vi "After Launch Init Core.vi"(8 "error in (no error)":errorcluster, 11 "CS++DeviceActor in":refnum<class "CS++DeviceActor.lvclass">) -> (0 "error out":errorcluster, 3 "CS++DeviceActor out":refnum<class "CS++DeviceActor.lvclass">)   [LabVIEW 2014, in "CS++DeviceActor.lvlib" / "CS++DeviceActor.lvclass"]
doc: "Use <b>Pre Launch init.vi</b> method for sanity checks that are supposed to prevent the actor from launching if they fail. Use <B>this</B> method instead to initialize this actor when it has been activated. A corresponding high priority message will become dispatched before the <B>Actor Core.vi</b> is called.\n\n<b>Derived classed should call the parent methode first</b> and their own initialization code after.\n\nRefer also to the ongoing discussion at https://decibel.ni.com/content/message/57394#57394."
uses:
  CS++DeviceActor.lvclass
  CS++DeviceActor.lvclass/CS++DeviceActor.ctl
  CS++BaseActor/CS++BaseActor.lvclass/CS++BaseActor.ctl
  <vilib>/ActorFramework/Actor/Actor.lvclass/Actor.ctl
  <vilib>/ActorFramework/Message Enqueuer/Message Enqueuer.lvclass/Message Enqueuer.ctl
  CS++DeviceActor Messages/Initialize Device Msg/Initialize Device Msg.lvclass/Initialize Device Msg.ctl
  CS++BaseActor Messages/Launch Associated GUI Msg/Launch Associated GUI Msg.lvclass/Launch Associated GUI Msg.ctl
  <vilib>/ActorFramework/Message Enqueuer/Enqueue.vi
  <vilib>/ActorFramework/Message Enqueuer/Init from Existing Queue.vi
  <vilib>/ActorFramework/Message Priority Queue/Priority Enqueue.vi
  CS++BaseActor/CS++BaseActor.lvclass
  CS++BaseActor Messages/Launch Associated GUI Msg/Launch Associated GUI Msg.lvclass
  CS++DeviceActor Messages/Selftest Device Msg/Selftest Device Msg.lvclass
  CS++DeviceActor Messages/Initialize Device Msg/Initialize Device Msg.lvclass
  <vilib>/ActorFramework/Message Enqueuer/Message Enqueuer.lvclass
  <vilib>/ActorFramework/Actor/Actor.lvclass
  Classes/CS++ProcessVariables/PVConnection/PVConnection.lvclass
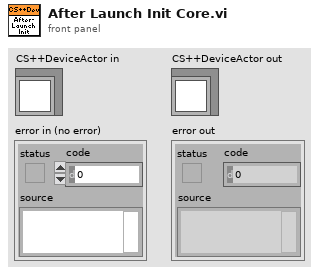
[diagram p1: front panel]
types:
  T1 = cluster{"Write Access":enum8{"Allowed", "Required", "None"}, "Read Access":enum8{"Allowed", "Required", "None"}}
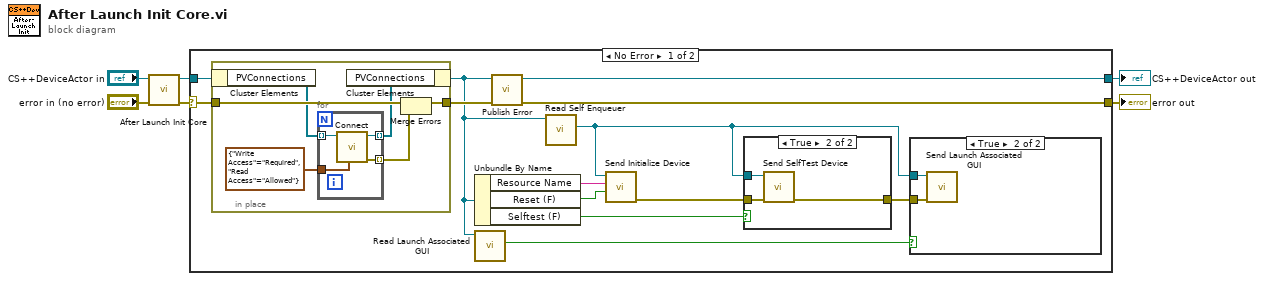
[diagram p0: block diagram]
diagram:
  n1 = call-parent "After Launch Init Core.vi"("error in (no error)"="error in (no error)", "CS++BaseActor in"="CS++DeviceActor in") -> ("error out"=w1:errorcluster, "CS++BaseActor out"=w3:refnum<class "CS++DeviceActor.lvclass">)  [unwired: 8 in]
  n2 = case shown="No Error" w1 {
    selector: w1 -> [w7 w36]
    tunnel: w3 -> [w8 w37]
    tunnel: [w11 w36] -> w6
    tunnel: [w10 w37] -> w5
    frame No Error {
      n3 = in-place {
        in-place-border: [w25] -> w18
        in-place-border: w7 -> [w24]
        n4 = in-place-cluster #1(w8) -> ("PVConnections"=w21:refnum<class "PVConnection.lvclass">[])
        n5 = for {
          tunnel: w21 -> [w29] mode=indexing
          tunnel: [w28] -> w20 mode=indexing
          tunnel: T1 {"Write Access"=enum."Required", "Read Access"=enum."Allowed"} ("Access") -> [w27]
          tunnel: [w26] -> w22 mode=indexing
          n6 = call "Connect.vi"("Access (R/W allowed)"=w27, "PVConnection in"=w29) -> ("error out"=w26:errorcluster, "PVConnection out"=w28:refnum<class "PVConnection.lvclass">)  [unwired: 8 in]
        }
        n7 = in-place-cluster #1("PVConnections"=w20) -> (w9:refnum<class "CS++DeviceActor.lvclass">)
        n8 = Merge Errors(w24, w22) -> (w25:errorcluster)
      }
      n9 = Unbundle By Name(w9) -> ("Resource Name"=w12:string, "Reset (F)"=w13:bool, "Selftest (F)"=w15:bool)
      n10 = call "Read Launch Associated GUI.vi"("CS++BaseActor in"=w9) -> ("Launch Associated GUI"=w19:bool)  [unwired: 8 in, 2 out]
      n11 = call "Publish Error.vi"("error in (no error)"=w18, "CS++DeviceActor in"=w9) -> ("error out"=w11:errorcluster, "CS++DeviceActor out"=w10:refnum<class "CS++DeviceActor.lvclass">)  [unwired: 8 in]
      n12 = call <vilib>:"Read Self Enqueuer.vi"("Actor"=w9) -> ("Self Enqueuer"=w16:refnum<class "Message Enqueuer.lvclass">)  [unwired: 10 in]
      n13 = call "Send Initialize Device.vi"("Reset (F)"=w13, "Resource Name"=w12, "Message Enqueuer"=w16) -> ("error out"=w14:errorcluster)  [unwired: 7 in, 1 out]
      n14 = case shown="True" w15 {
        tunnel: w16 -> [_ w35]
        tunnel: w14 -> [w32 w34]
        tunnel: [w32 w33] -> w17
        frame False {
        }
        frame True {
          n15 = call "Send SelfTest Device.vi"("error in (no error)"=w34, "Message Enqueuer"=w35) -> ("error out"=w33:errorcluster)  [unwired: 8 in, 1 out]
        }
      }
      n16 = case shown="True" w19 {
        tunnel: w16 -> [_ w31]
        tunnel: w17 -> [_ w30]
        frame False {
        }
        frame True {
          n17 = call "Send Launch Associated GUI.vi"("error in (no error)"=w30, "Message Enqueuer"=w31) -> ()  [unwired: 8 in, 2 out]
        }
      }
    }
    frame Error {
    }
  }
  "error out" <- w6
  "CS++DeviceActor out" <- w5
